vi "AngleCycle.vi"(7 "MAX":sgl, 10 "Angle":sgl) -> (2 "AngleOut":sgl)   [LabVIEW 2015]
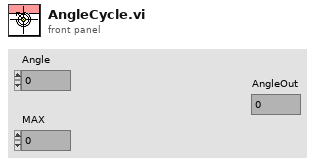
[diagram p1: front panel]
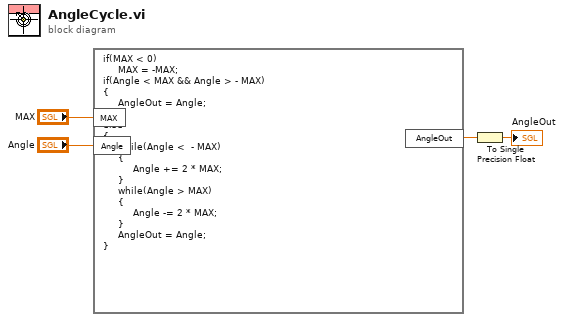
[diagram p0: block diagram]
diagram:
  n1 = formula code="if(MAX < 0)\n     MAX = -MAX;\nif(Angle < MAX && Angle > - MAX)\n{\n     AngleOut = Angle;\n}\nelse\n{\n     while(Angle <  - MAX)\n     {\n          Angle += 2 * MAX;\n     }\n     while(Angle > MAX)\n     {\n          Angle -= 2 * MAX;\n     }\n     AngleOut = Angle;\n}"("MAX"="MAX", "Angle"="Angle") -> ("AngleOut"=w1:dbl)
  n2 = To Single Precision Float(number=w1) -> (single precision float=→"AngleOut":sgl)
